vi "Config CDMA2000 Reverse.vi"(0 "VISA Resource Name":refnum<visa-resource-name>, 1 "Forward Select (3: S1 9 Channel)":T2(ring)=enum."S3 5 Channel", 2 "Custom State File (CDMA_DATA)":string="CDMA_DATA", 4 "Reconstruction Filter (1: 2.5MHZ)":T1(ring)=enum."2.5 MHZ", 5 "error in (no error)":errorcluster {"code" format="%.0x"}, 10 "ARB Reference (F:INT)":bool, 12 "Reference Freq (10.0)":dbl=10.0 format="%.8f") -> (14 "VISA Resource Name Out":refnum<visa-resource-name>, 19 "error out":errorcluster {"code" format="%.0x"})   [LabVIEW 2014, in "Agilent ESG Series.lvlib"]
doc: "This VI is used to configure the reverse CDMA2000 option.\n\nNotes:\nThis VI is valid only on instruments E44xxB with the 101 option or on instrument E4438C with option 401."
uses:
  Agilent ESG Series.lvlib
panel:
  # "EXT"
  # "INT"
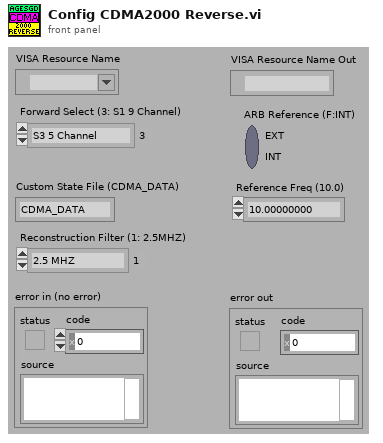
[diagram p1: front panel]
types:
  T1 = enum16{"250 KHZ", "2.5 MHZ", "8.0 MHZ", "THROUGH"}
  T2 = enum16{"S1 Pilot", "S3 Pilot", "S1 5 Channel", "S3 5 Channel", "S1 8 Channel", "Custom"}
  T3 = enum16{"PILOT", "9 CH FWD", "32 CH FWD", "64 CH FWD", "REVERSE", "CUSTOM"}
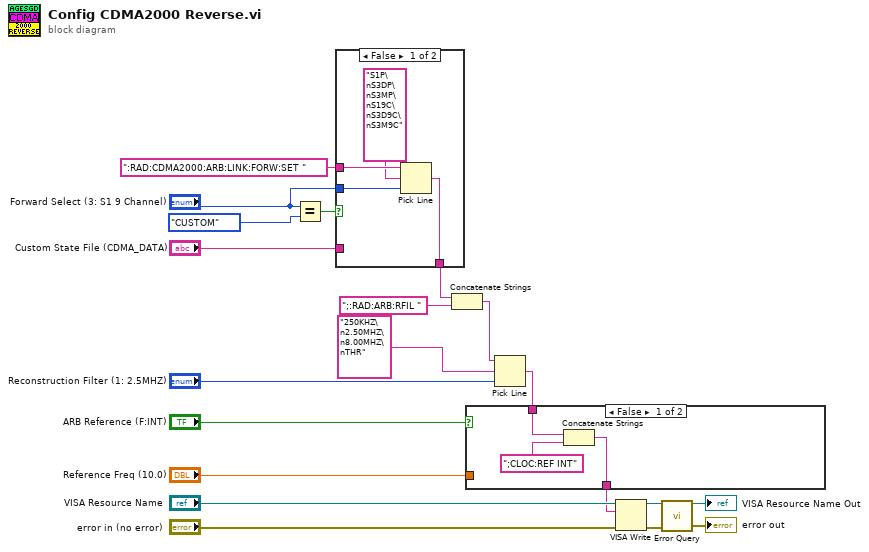
[diagram p0: block diagram]
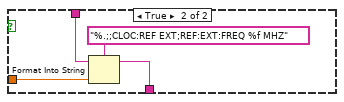
[diagram p2: hidden frame]
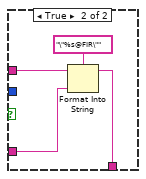
[diagram p3: hidden frame]
diagram:
  n1 = Equal?(x="Forward Select (3: S1 9 Channel)", y=T3."CUSTOM") -> (x = y?=w17:bool)
  n2 = case shown="False" w17 {
    tunnel: ":RAD:CDMA2000:ARB:LINK:FORW:SET " ("string (\"\")") -> [w24 w28]
    tunnel: "Forward Select (3: S1 9 Channel)" -> [w22 _]
    tunnel: [w21 w26] -> w1
    tunnel: "Custom State File (CDMA_DATA)" -> [_ w25]
    frame False {
      n3 = Pick Line(string ("")=w24, multi-line string="S1P\nS3DP\nS3MP\nS19C\nS3D9C\nS3M9C", line index=w22) -> (output string=w21:string)
    }
    frame True {
      n4 = Format Into String(format string="\"%s@FIR\"", initial string=w28, w25) -> (resulting string=w26:string)  [unwired: 1 in, 1 out]
    }
  }
  n5 = Concatenate Strings(w1, ";:RAD:ARB:RFIL " ("string (\"\")")) -> (w10:string)
  n6 = Pick Line(string ("")=w10, multi-line string="250KHZ\n2.50MHZ\n8.00MHZ\nTHR", line index="Reconstruction Filter (1: 2.5MHZ)") -> (output string=w11:string)
  n7 = case shown="False" "ARB Reference (F:INT)" {
    tunnel: w11 -> [w31 w35]
    tunnel: [w29 w32] -> w6
    tunnel: "Reference Freq (10.0)" -> [_ w33]
    frame False {
      n8 = Concatenate Strings(w31, ";CLOC:REF INT") -> (w29:string)
    }
    frame True {
      n9 = Format Into String(format string="%.;;CLOC:REF EXT;REF:EXT:FREQ %f MHZ", initial string=w35, w33) -> (resulting string=w32:string)  [unwired: 1 in, 1 out]
    }
  }
  n10 = VISA Write(VISA resource name="VISA Resource Name", write buffer=w6, error in (no error)="error in (no error)") -> (VISA resource name out=w5:refnum<visa-resource-name>, error out=w4:errorcluster)  [unwired: 1 out]
  n11 = call "Error Query.vi"("VISA Resource Name"=w5, "error in (no error)"=w4) -> ("VISA Resource Name Out"=→"VISA Resource Name Out":refnum<visa-resource-name>, "error out"=→"error out":errorcluster)  [unwired: 10 in, 2 out]
